vi "GetExposure.vi"(8 "error in":errorcluster, 11 "camera.nit_c in":refnum<class "camera.lvclass">) -> (0 "error out":errorcluster, 2 "exposure":dbl)   [LabVIEW 2020, in "camera.lvclass"]
uses:
  camera.lvclass
  camera.lvclass/camera.ctl
  lib/O-PL.dll
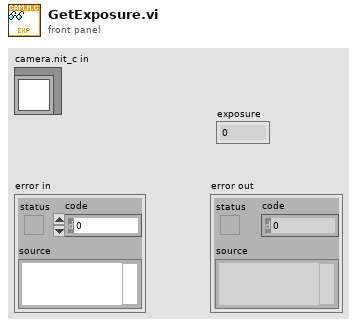
[diagram p1: front panel]
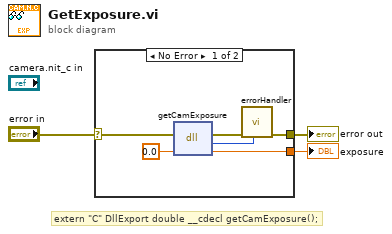
[diagram p0: block diagram]
diagram:
  # "extern \"C\" DllExport double __cdecl getCamExposure();"
  n1 = case shown="No Error" "error in" {
    selector: "error in" -> [w9 _]
    tunnel: [w4 _] -> w3
    tunnel: [w7 _] -> w2
    frame No Error {
      n2 = dll-call lib="D:/UNSW - New/v0.8.3/lib/O-PL.dll" fn="getCamExposure"(error in=w9, "exposure"=0.0) -> (error out=w6:errorcluster, "return type"=w5:i32, "exposure"=w7:dbl)  [unwired: 2 in, 1 out]
      n3 = call "errorHandler.vi"("code"=w5, "error in"=w6) -> ("error out"=w4:errorcluster)  [unwired: 9 in]
    }
    frame Error {
    }
  }
  "error out" <- w3
  "exposure" <- w2
